vi "User Shell EOD reader.vi"() -> ()   [LabVIEW 2014]
panel:
  out "output cluster":T1
  in  "file path (use dialog)":path
  in  "Exit":bool
  in  "Run":bool
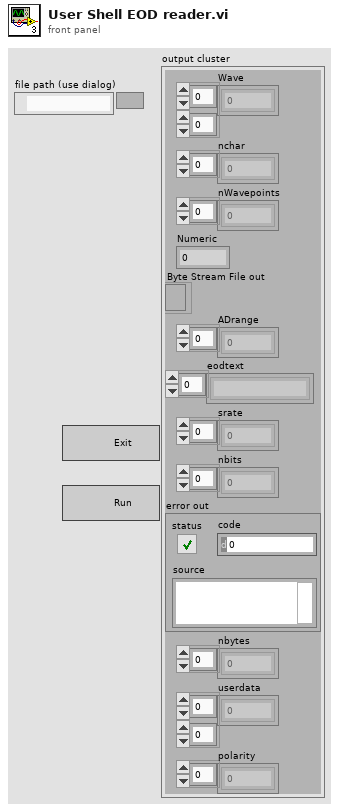
[diagram p1: front panel]
types:
  T1 = cluster{"Wave":i16[][], "nchar":u8[], "nWavepoints":u32[], "Numeric":i32, "Byte Stream File out":refnum<file>, "ADrange":sgl[], "eodtext":string[], "srate":u32[], "nbits":i8[], "error out":errorcluster, "nbytes":i8[], "userdata":sgl[][], "polarity":i8[]}
  T2 = enum16{"Run", "Wait", "Change value", "Exit", "Display message"}
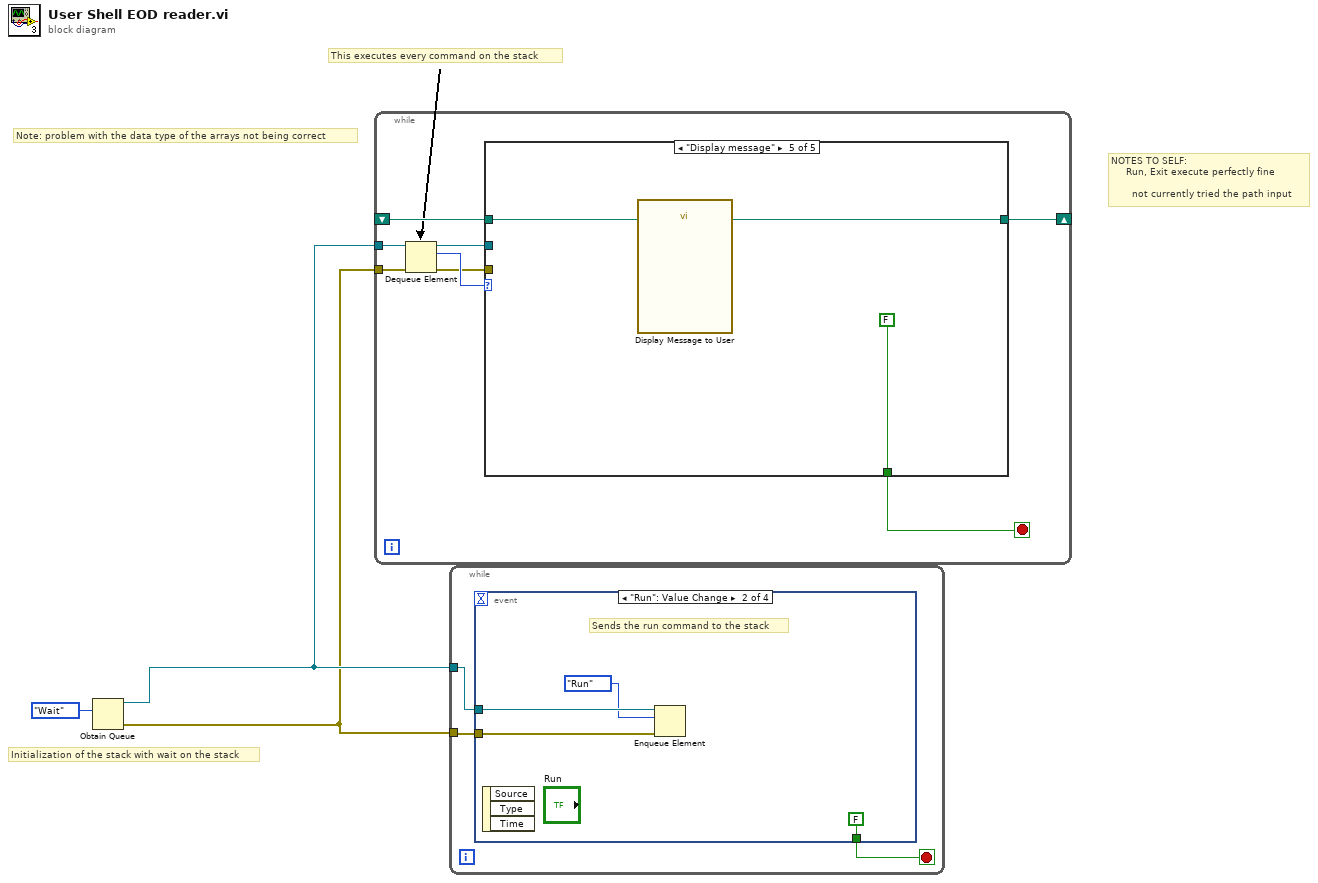
[diagram p0: block diagram]
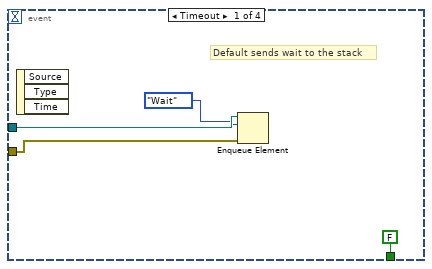
[diagram p2: hidden frame]
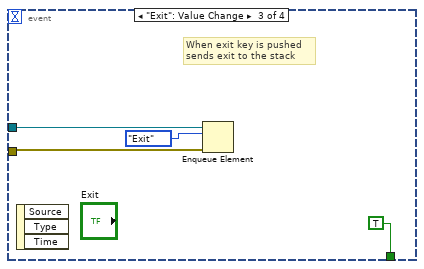
[diagram p3: hidden frame]
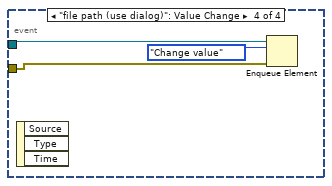
[diagram p4: hidden frame]
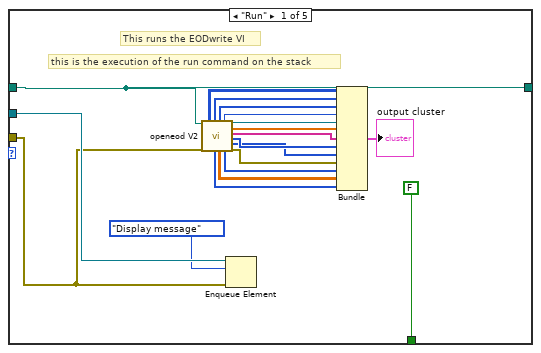
[diagram p5: hidden frame]
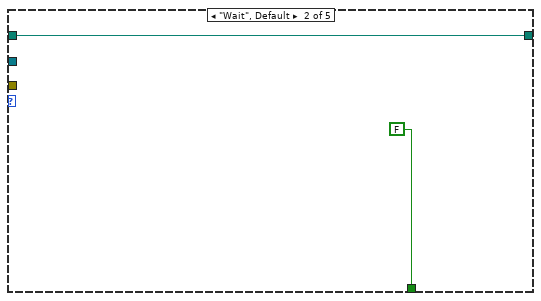
[diagram p6: hidden frame]
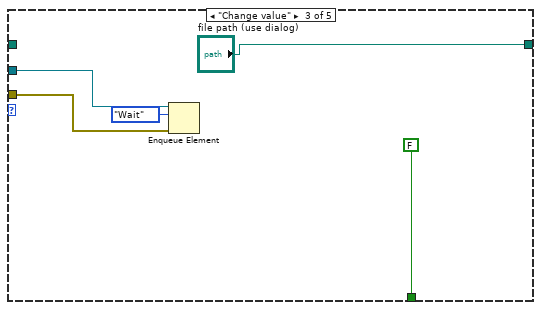
[diagram p7: hidden frame]
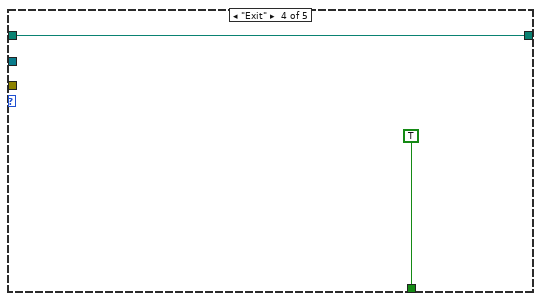
[diagram p8: hidden frame]
diagram:
  # "NOTES TO SELF:\n     Run, Exit execute perfectly fine\n\n       not currently tried the path input"
  # "Initialization of the stack with wait on the stack"
  # "This executes every command on the stack"
  # "Note: problem with the data type of the arrays not being correct"
  n1 = Obtain Queue(element data type=T2."Wait") -> (queue out=w2:refnum<queue>, error out=w1:errorcluster)  [unwired: 4 in, 1 out]
  n2 = while {
    tunnel: w2 -> [w10]
    tunnel: w1 -> [w9]
    shift-right: [w7] -> _
    shift-left: _ -> [w6]
    stop <- w11 stop-if-true
    n3 = Dequeue Element(queue=w10, error in (no error)=w9) -> (queue out=w5:refnum<queue>, element=w8:T2, error out=w4:errorcluster)  [unwired: 1 in, 1 out]
    n4 = case shown="\"Display message\"" w8 {
      tunnel: [FALSE FALSE FALSE TRUE FALSE] -> w11
      tunnel: [w13 w31 "file path (use dialog)" w38 w40] -> w7
      tunnel: w6 -> [w13 w31 _ w38 w40]
      tunnel: w5 -> [w29 _ w35 _ _]
      tunnel: w4 -> [w12 _ w34 _ _]
      frame "Run" {
        # "this is the execution of the run command on the stack"
        # "This runs the EODwrite VI"
        n5 = call "openeod V2.vi"("file path"=w13, "error in (no error)"=w12) -> ("Wave"=w27:i16[][], "nchar"=w26:u8[], "polarity"=w15:i8[], "nWavepoints"=w25:u32[], "userdata"=w16:sgl[][], "Numeric"=w24:i32, "nbytes"=w17:i8[], "Byte Stream File out"=w23:refnum<file>, "ADrange"=w22:sgl[], "eodtext"=w21:string[], "srate"=w20:u32[], "nbits"=w19:i8[], "error out"=w18:errorcluster)  [unwired: 5 in]
        n6 = Enqueue Element(queue=w29, element=T2."Display message", error in (no error)=w12) -> ()  [unwired: 1 in, 3 out]
        n7 = Bundle("Wave"=w27, "nchar"=w26, "nWavepoints"=w25, "Numeric"=w24, "Byte Stream File out"=w23, "ADrange"=w22, "eodtext"=w21, "srate"=w20, "nbits"=w19, "error out"=w18, "nbytes"=w17, "userdata"=w16, "polarity"=w15) -> (→"output cluster":T1)  [unwired: 1 in]
      }
      frame "Wait", Default {
      }
      frame "Change value" {
        n8 = Enqueue Element(queue=w35, element=T2."Wait", error in (no error)=w34) -> ()  [unwired: 1 in, 3 out]
      }
      frame "Exit" {
      }
      frame "Display message" {
        n9 = call "Display Message to User"() -> ()  [unwired: 10 in, 2 out]
      }
    }
  }
  n10 = while {
    tunnel: w2 -> [w44]
    tunnel: w1 -> [w43]
    stop <- w42 stop-if-true
    n11 = event shown="[1] \"Run\": Value Change" {
      selector: _ -> [_ _ _ _]
      dyn-events: _ -> [_ _ _ _]
      timeout: _ -> [_ _ _ _]
      tunnel: w44 -> [w48 w52 w55 w58]
      tunnel: w43 -> [w47 w51 w54 w57]
      tunnel: [FALSE FALSE TRUE _] -> w42
      event Timeout {
        # "Default sends wait to the stack"
        n12 = event-data() -> ()  [unwired: 1 in, 3 out]
        n13 = Enqueue Element(queue=w48, element=T2."Wait", error in (no error)=w47) -> ()  [unwired: 1 in, 3 out]
      }
      event "Run": Value Change {
        # "Sends the run command to the stack"
        n14 = event-data() -> ()  [unwired: 1 in, 3 out]
        n15 = Enqueue Element(queue=w52, element=T2."Run", error in (no error)=w51) -> ()  [unwired: 1 in, 3 out]
      }
      event "Exit": Value Change {
        # "When exit key is pushed\nsends exit to the stack"
        n16 = event-data() -> ()  [unwired: 1 in, 3 out]
        n17 = Enqueue Element(queue=w55, element=T2."Exit", error in (no error)=w54) -> ()  [unwired: 1 in, 3 out]
      }
      event "file path (use dialog)": Value Change {
        n18 = event-data() -> ()  [unwired: 1 in, 3 out]
        n19 = Enqueue Element(queue=w58, element=T2."Change value", error in (no error)=w57) -> ()  [unwired: 1 in, 3 out]
      }
    }
  }
